vi "Get Parameters Values.vi"(8 "error in (no error)":errorcluster, 11 "Run Optimiser in":refnum<class "Optimiser Cell.lvclass">) -> (0 "error out":errorcluster, 2 "Optimisation Parameters":T1[](array[typedef]), 3 "Run Optimiser out":refnum<class "Optimiser Cell.lvclass">)   [LabVIEW 2020, in "Run Utilities.lvlib" / "Optimiser Cell.lvclass"]
uses:
  Optimiser Cell.lvclass
  Name with value pair.ctl
  Optimiser Cell.lvclass/Optimiser Cell.ctl
  Analysis Framework/Analysis Framework.lvclass
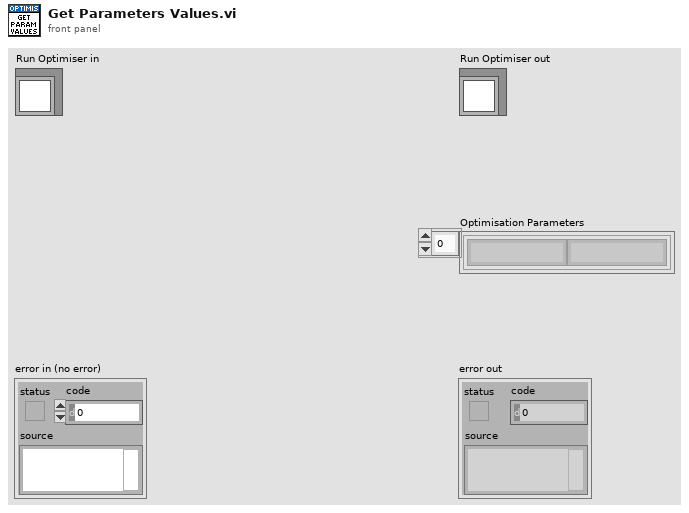
[diagram p1: front panel]
types:
  T1 = typedef "Analysis Framework.lvclass/Name with value pair.ctl" = cluster{"Name":string, "Value":string}
  T2 = typedef "Run Utilities.lvlib/Optimiser Cell.lvclass/Optimise parameter - numeric.ctl" = cluster{"Name":string, "Start value":dbl, "From":dbl, "To":dbl, "dtype":enum16{"INT", "DBL"}}
  T3 = typedef "Run Utilities.lvlib/Optimiser Cell.lvclass/Optimise parameter - string.ctl" = cluster{"Name":string, "Start value":string, "Options":string[]}
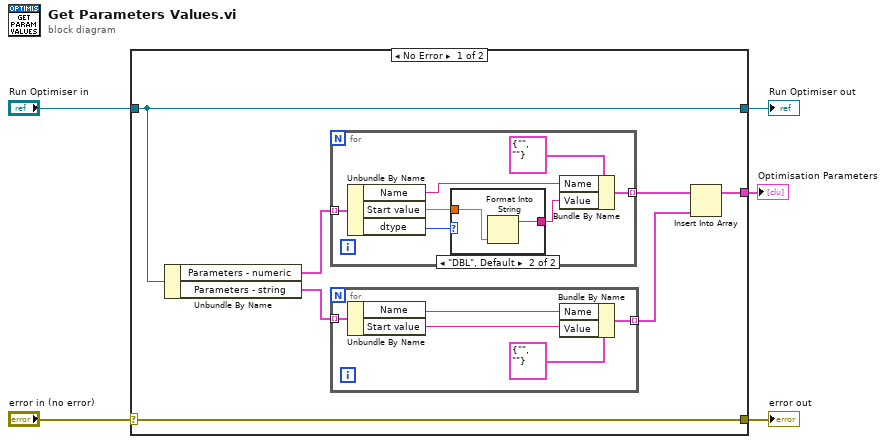
[diagram p0: block diagram]
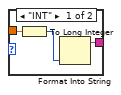
[diagram p2: hidden frame]
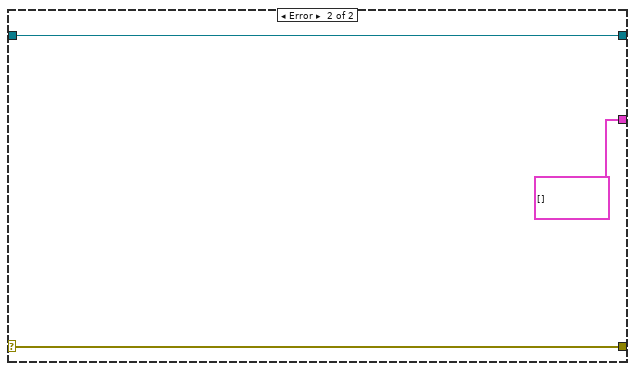
[diagram p3: hidden frame]
diagram:
  n1 = case shown="No Error" "error in (no error)" {
    selector: "error in (no error)" -> [w12 w32]
    tunnel: [w12 w32] -> w4
    tunnel: [w11 w31] -> w2
    tunnel: "Run Optimiser in" -> [w11 w31]
    tunnel: [w7 T1[] []] -> w1
    frame No Error {
      n2 = Unbundle By Name(w11) -> ("Parameters - numeric"=w10:T2[], "Parameters - string"=w9:T3[])
      n3 = for {
        tunnel: w10 -> [w24] mode=indexing
        tunnel: [w18] -> w8 mode=indexing
        n4 = Unbundle By Name(w24) -> ("Name"=w19:string, "Start value"=w22:dbl, "dtype"=w23:enum16{"INT", "DBL"})
        n5 = case shown="\"DBL\", Default" w23 {
          tunnel: w22 -> [w27 w29]
          tunnel: [w25 w28] -> w20
          frame "INT" {
            n6 = To Long Integer(number=w27) -> (32bit integer=w26:i32)
            n7 = Format Into String(w26) -> (resulting string=w25:string)  [unwired: 3 in, 1 out]
          }
          frame "DBL", Default {
            n8 = Format Into String(w29) -> (resulting string=w28:string)  [unwired: 3 in, 1 out]
          }
        }
        n9 = Bundle By Name(cluster=T1 {"Name"="", "Value"=""} ("Parameter"), "Name"=w19, "Value"=w20) -> (w18:T1)
      }
      n10 = for {
        tunnel: w9 -> [w17] mode=indexing
        tunnel: [w13] -> w6 mode=indexing
        n11 = Unbundle By Name(w17) -> ("Name"=w15:string, "Start value"=w14:string)
        n12 = Bundle By Name(cluster=T1 {"Name"="", "Value"=""} ("Parameter"), "Name"=w15, "Value"=w14) -> (w13:T1)
      }
      n13 = Insert Into Array(array=w8, new element=w6) -> (w7:T1[])  [unwired: 1 in]
    }
    frame Error {
    }
  }
  "error out" <- w4
  "Run Optimiser out" <- w2
  "Optimisation Parameters" <- w1
